vi "Short segment creater.vi"(8 "deltaX":dbl, 9 "Velocity":dbl, 10 "Time Period":dbl, 11 "LastTimeSegment":T1) -> (3 "TimeSegment out":T1)   [LabVIEW 2014]
uses:
  TimeSegment.ctl
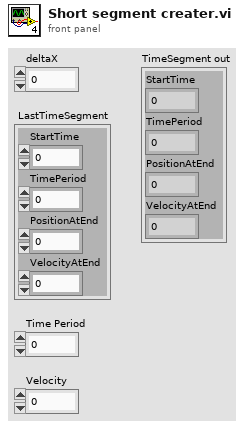
[diagram p1: front panel]
types:
  T1 = typedef "TimeSegment.ctl" = cluster{"StartTime":dbl, "TimePeriod":dbl, "PositionAtEnd":dbl, "VelocityAtEnd":dbl}
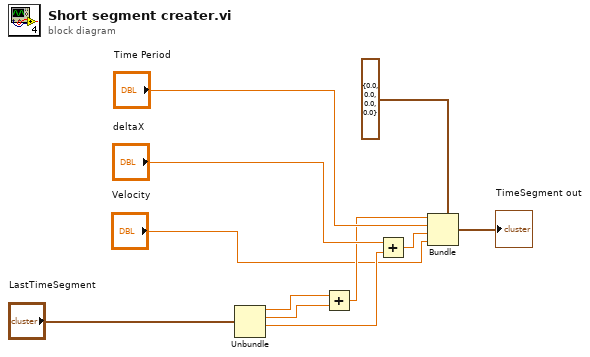
[diagram p0: block diagram]
diagram:
  n1 = Unbundle("LastTimeSegment") -> ("StartTime"=w3:dbl, "TimePeriod"=w4:dbl, "PositionAtEnd"=w8:dbl)  [unwired: 1 out]
  n2 = Add(x=w3, y=w4) -> (x+y=w2:dbl)
  n3 = Add(x="deltaX", y=w8) -> (x+y=w10:dbl)
  n4 = Bundle(cluster=T1 {"StartTime"=0.0, "TimePeriod"=0.0, "PositionAtEnd"=0.0, "VelocityAtEnd"=0.0} ("TimeSegment"), "StartTime"=w2, "TimePeriod"="Time Period", "PositionAtEnd"=w10, "VelocityAtEnd"="Velocity") -> (→"TimeSegment out":T1)
